vi "GFITS_CollectHeaders.vi"(2 "Database RefNum in":T1, 7 "Keywords":string[][](array[string]), 9 "extension":i16=-1, 11 "error in (no error)":errorcluster, 13 "nd queue":bool) -> (8 "headers":string[][](table), 15 "error out":errorcluster)   [LabVIEW 2016]
uses:
  GFITS_datatypesctl.ctl
  DBSHAND/private/vis/DatabaseHand_RefNum.ctl
panel:
  in  "Types":T2={"TBIT"=1, "TBYTE"=11, "TSTRING"=16, "TSHORT"=21, "TLONG"=41, "TFLOAT"=42, "TDOUBLE"=82, "TCOMPLEX"=83, "TDBLCOMPLEX"=163, "TUINT"=30, "TUSHORT"=20, "TULONG"=40, "TINT"=31, "TSBYTE"=12, "TLONGLONG"=81, "TLOGICAL"=14}
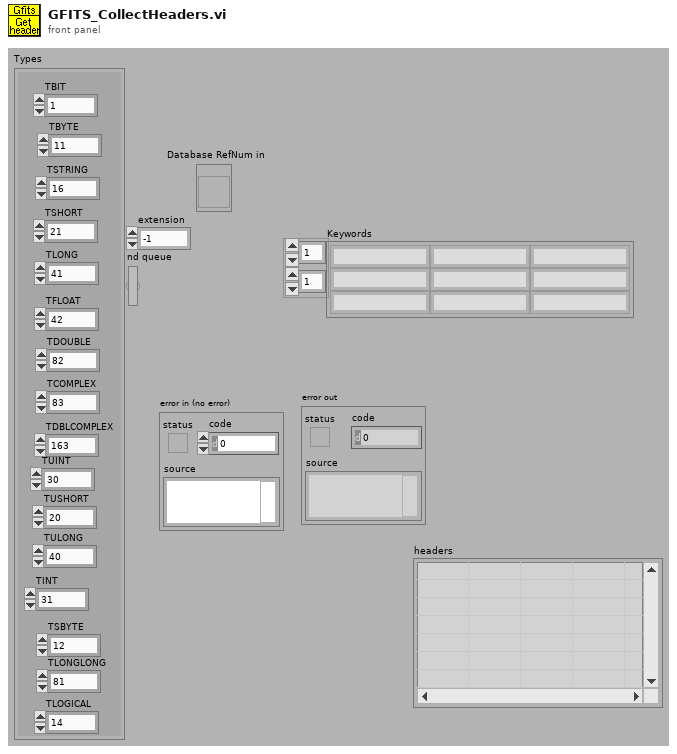
[diagram p1: front panel]
types:
  T1 = typedef "DatabaseHand_RefNum.ctl" = refnum<vi>
  T2 = typedef "GFITS_datatypesctl.ctl" = cluster{"TBIT":i32, "TBYTE":i32, "TSTRING":i32, "TSHORT":i32, "TLONG":i32, "TFLOAT":i32, "TDOUBLE":i32, "TCOMPLEX":i32, "TDBLCOMPLEX":i32, "TUINT":i32, "TUSHORT":i32, "TULONG":i32, "TINT":i32, "TSBYTE":i32, "TLONGLONG":i32, "TLOGICAL":i32}
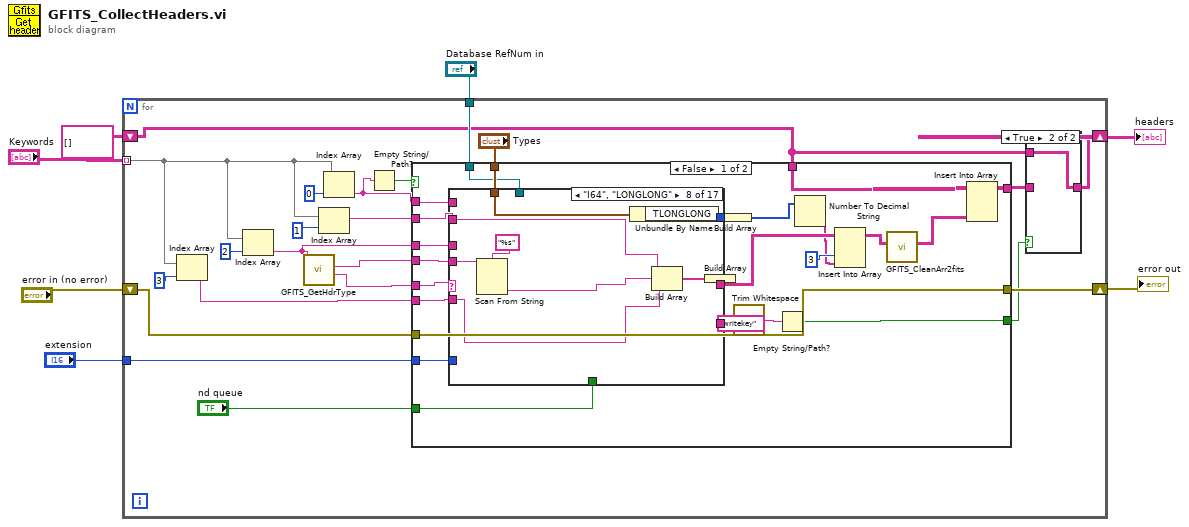
[diagram p0: block diagram]
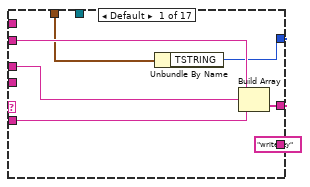
[diagram p3: hidden frame]
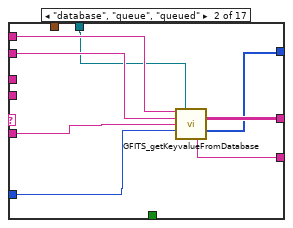
[diagram p4: hidden frame]
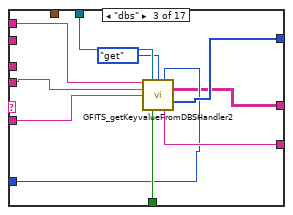
[diagram p5: hidden frame]
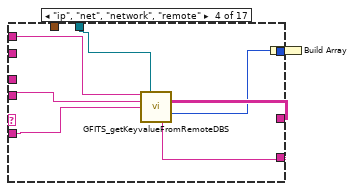
[diagram p6: hidden frame]
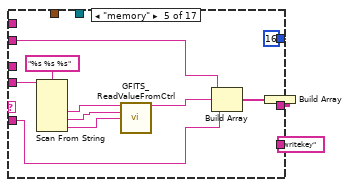
[diagram p7: hidden frame]
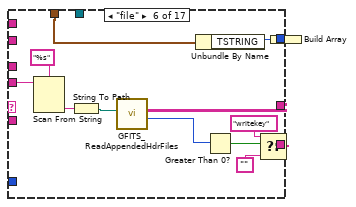
[diagram p8: hidden frame]
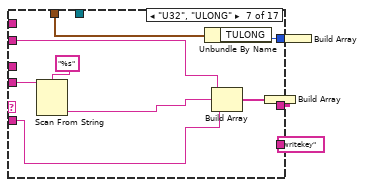
[diagram p9: hidden frame]
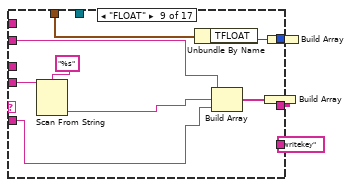
[diagram p10: hidden frame]
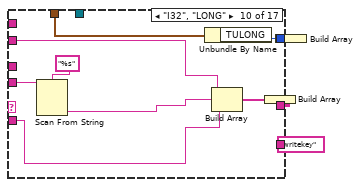
[diagram p11: hidden frame]
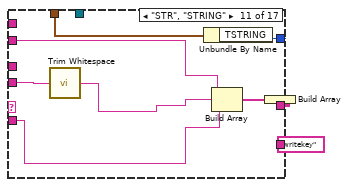
[diagram p12: hidden frame]
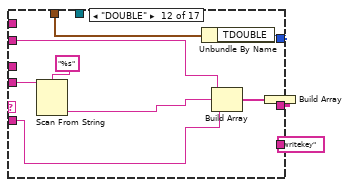
[diagram p13: hidden frame]
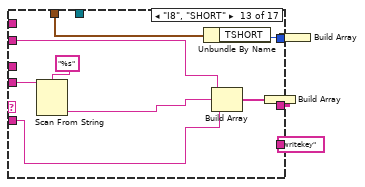
[diagram p14: hidden frame]
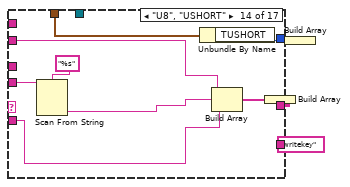
[diagram p15: hidden frame]
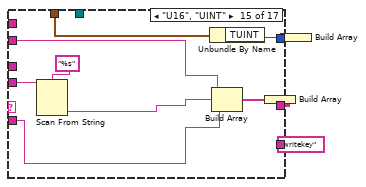
[diagram p16: hidden frame]
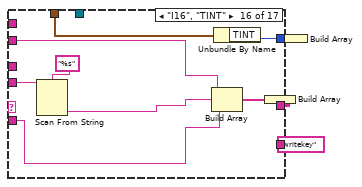
[diagram p17: hidden frame]
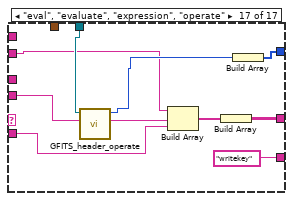
[diagram p18: hidden frame]
diagram:
  n1 = for {
    tunnel: "Keywords" -> [w24] mode=indexing
    shift-right: [w15] -> w6
    shift-left: "error in (no error)" -> [w19]
    tunnel: "Database RefNum in" -> [w18]
    shift-right: [w9] -> w2
    shift-left: string[][] [] -> [w8]
    tunnel: "extension" -> [w13]
    n2 = Index Array(array=w24, index=3 ("Array Index")) -> (element=w25:string)
    n3 = Index Array(array=w24, index=2 ("Array Index")) -> (element=w14:string)
    n4 = call "GFITS_GetHdrType.vi"("keyval"=w14) -> ("type"=w17:string, "keyval out"=w16:string)  [unwired: 9 out]
    n5 = Index Array(array=w24, index=1 ("Array Index")) -> (element=w26:string)
    n6 = Index Array(array=w24, index=0 ("Index")) -> (element=w22:string)
    n7 = Empty String/Path?(string/path=w22) -> (empty?=w21:bool)
    n8 = case shown="False" w21 {
      selector: w21 -> [_ w234]
      tunnel: w26 -> [w52 _]
      tunnel: w25 -> [w49 _]
      tunnel: w17 -> [w50 _]
      tunnel: w16 -> [w51 _]
      tunnel: w22 -> [w53 _]
      tunnel: "Types" -> [w48 _]
      tunnel: [w46 w236] -> w15
      tunnel: w19 -> [w46 w236]
      tunnel: w18 -> [w47 _]
      tunnel: [w45 w235] -> w10
      tunnel: w8 -> [w44 w235]
      tunnel: w14 -> [w43 _]
      tunnel: w13 -> [w38 _]
      tunnel: "nd queue" -> [w37 _]
      tunnel: [w34 w234] -> w11
      frame False {
        n9 = case shown="\"I64\", \"LONGLONG\"" w50 {
          tunnel: w49 -> [w60 w69 w77 w83 w93 _ w121 w132 w143 w154 w166 w175 w186 w197 w208 w219 w227]
          tunnel: ["writekey" w70 w76 w88 "writekey" ("function to use") w103 "writekey" ("function to use") "writekey" ("function to use") "writekey" ("function to use") "writekey" ("function to use") "writekey" ("function to use") "writekey" ("function to use") "writekey" ("function to use") "writekey" ("function to use") "writekey" ("function to use") "writekey" ("function to use") "writekey" ("function to use")] -> w36
          tunnel: [w57 w64 w74 w81 w89 w102 w115 w126 w137 w148 w159 w169 w180 w191 w202 w213 w225] -> w40
          tunnel: w52 -> [w61 w66 _ _ w94 _ w122 w133 w144 w155 w167 w176 w187 w198 w209 w220 w226]
          tunnel: w51 -> [_ _ w78 w84 w101 w112 w125 w136 w147 w158 w161 w179 w190 w201 w212 w223 w230]
          tunnel: [w58 w68 w71 w87 w90 w106 w119 w130 w141 w152 w164 w173 w184 w195 w206 w217 w228] -> w42
          tunnel: w53 -> [_ w67 w79 w85 _ _ _ _ _ _ _ _ _ _ _ _ _]
          tunnel: w48 -> [w56 _ _ _ _ w114 w117 w128 w139 w150 w163 w171 w182 w193 w204 w215 _]
          tunnel: w47 -> [_ w65 w80 w82 _ _ _ _ _ _ _ _ _ _ _ _ w229]
          tunnel: w43 -> [w54 _ _ _ _ _ _ _ _ _ _ _ _ _ _ _ _]
          tunnel: w38 -> [_ w63 w72 _ _ _ _ _ _ _ _ _ _ _ _ _ _]
          tunnel: w37 -> [_ _ w73 _ _ _ _ _ _ _ _ _ _ _ _ _ _]
          frame Default {
            n10 = Unbundle By Name(w56) -> ("TSTRING"=w55:i32)
            n11 = Build Array(w61, w54, w60) -> (w59:string[])
            n12 = Build Array(w55) -> (w57:i32[])
            n13 = Build Array(w59) -> (w58:string[][])
          }
          frame "database", "queue", "queued" {
            n14 = call "GFITS_getKeyvalueFromDatabase.vi"("key name in header"=w67, "Database RefNum in"=w65, "Keyname"=w66, "comment"=w69, "extension"=w63) -> ("table out"=w68:string[][], "datatype"=w64:u16[], "function to use"=w70:string)  [unwired: 1 in, 7 out]
          }
          frame "dbs" {
            n15 = call "GFITS_getKeyvalueFromDBSHandler2.vi"("key name in header"=w79, "Database RefNum in"=w80, "action"=enum16{"get", "clear"}."get", "extension"=w72, "varname"=w78, "comment"=w77, "nd queue"=w73) -> ("table out"=w71:string[][], "datatype"=w74:u16[], "function to use"=w76:string)  [unwired: 2 in, 4 out]
          }
          frame "ip", "net", "network", "remote" {
            n16 = call "GFITS_getKeyvalueFromRemoteDBS.vi"("key name in header"=w85, "Database RefNum in"=w82, "varname"=w84, "comment"=w83) -> ("table out"=w87:string[][], "datatype"=w86:u16, "function to use"=w88:string)  [unwired: 2 in, 7 out]
            n17 = Build Array(w86) -> (w81:u16[])
          }
          frame "memory" {
            n18 = Scan From String(format string="%s %s %s" ("Format String"), input string=w101) -> (output 1=w99:string, output 2=w98:string, output 3=w97:string)  [unwired: 2 in, 6 out]
            n19 = call "GFITS_ReadValueFromCtrl.vi"("Vi name"=w99, "Control Name"=w98, "Type"=w97) -> ("Value"=w92:string)  [unwired: 1 in, 11 out]
            n20 = Build Array(w94, w92, w93) -> (w91:string[])
            n21 = Build Array(w91) -> (w90:string[][])
            n22 = Build Array(16 ("datatype")) -> (w89:i32[])
          }
          frame "file" {
            n23 = Scan From String(format string="%s", input string=w112) -> (output 1=w110:string)  [unwired: 2 in, 4 out]
            n24 = String To Path(string=w110) -> (path=w109:path)
            n25 = call "GFITS_ReadAppendedHdrFiles.vi"("Path"=w109) -> ("keywords found"=w108:i32, "Array"=w106:string[][])  [unwired: 1 in, 8 out]
            n26 = Unbundle By Name(w114) -> ("TSTRING"=w113:i32)
            n27 = Greater Than 0?(x=w108) -> (x > 0?=w107:bool)
            n28 = Select(t="writekey" ("function to use"), s=w107, f="") -> (s? t:f=w103:string)
            n29 = Build Array(w113) -> (w102:i32[])
          }
          frame "U32", "ULONG" {
            n30 = Scan From String(format string="%s" ("Format String"), input string=w125) -> (output 1=w118:string)  [unwired: 2 in, 4 out]
            n31 = Unbundle By Name(w117) -> ("TULONG"=w116:i32)
            n32 = Build Array(w122, w118, w121) -> (w120:string[])
            n33 = Build Array(w120) -> (w119:string[][])
            n34 = Build Array(w116) -> (w115:i32[])
          }
          frame "I64", "LONGLONG" {
            n35 = Scan From String(format string="%s" ("Format String"), input string=w136) -> (output 1=w129:string)  [unwired: 2 in, 4 out]
            n36 = Unbundle By Name(w128) -> ("TLONGLONG"=w127:i32)
            n37 = Build Array(w133, w129, w132) -> (w131:string[])
            n38 = Build Array(w131) -> (w130:string[][])
            n39 = Build Array(w127) -> (w126:i32[])
          }
          frame "FLOAT" {
            n40 = Scan From String(format string="%s" ("Format String"), input string=w147) -> (output 1=w140:string)  [unwired: 2 in, 4 out]
            n41 = Unbundle By Name(w139) -> ("TFLOAT"=w138:i32)
            n42 = Build Array(w144, w140, w143) -> (w142:string[])
            n43 = Build Array(w142) -> (w141:string[][])
            n44 = Build Array(w138) -> (w137:i32[])
          }
          frame "I32", "LONG" {
            n45 = Scan From String(format string="%s" ("Format String"), input string=w158) -> (output 1=w151:string)  [unwired: 2 in, 4 out]
            n46 = Unbundle By Name(w150) -> ("TULONG"=w149:i32)
            n47 = Build Array(w155, w151, w154) -> (w153:string[])
            n48 = Build Array(w153) -> (w152:string[][])
            n49 = Build Array(w149) -> (w148:i32[])
          }
          frame "STR", "STRING" {
            n50 = call <vilib>:"Trim Whitespace.vi"("string"=w161) -> ("trimmed string"=w160:string)  [unwired: 1 in]
            n51 = Unbundle By Name(w163) -> ("TSTRING"=w162:i32)
            n52 = Build Array(w167, w160, w166) -> (w165:string[])
            n53 = Build Array(w165) -> (w164:string[][])
            n54 = Build Array(w162) -> (w159:i32[])
          }
          frame "DOUBLE" {
            n55 = Scan From String(format string="%s" ("Format String"), input string=w179) -> (output 1=w172:string)  [unwired: 2 in, 4 out]
            n56 = Unbundle By Name(w171) -> ("TDOUBLE"=w170:i32)
            n57 = Build Array(w176, w172, w175) -> (w174:string[])
            n58 = Build Array(w174) -> (w173:string[][])
            n59 = Build Array(w170) -> (w169:i32[])
          }
          frame "I8", "SHORT" {
            n60 = Scan From String(format string="%s" ("Format String"), input string=w190) -> (output 1=w183:string)  [unwired: 2 in, 4 out]
            n61 = Unbundle By Name(w182) -> ("TSHORT"=w181:i32)
            n62 = Build Array(w187, w183, w186) -> (w185:string[])
            n63 = Build Array(w185) -> (w184:string[][])
            n64 = Build Array(w181) -> (w180:i32[])
          }
          frame "U8", "USHORT" {
            n65 = Scan From String(format string="%s" ("Format String"), input string=w201) -> (output 1=w194:string)  [unwired: 2 in, 4 out]
            n66 = Unbundle By Name(w193) -> ("TUSHORT"=w192:i32)
            n67 = Build Array(w198, w194, w197) -> (w196:string[])
            n68 = Build Array(w196) -> (w195:string[][])
            n69 = Build Array(w192) -> (w191:i32[])
          }
          frame "U16", "UINT" {
            n70 = Scan From String(format string="%s" ("Format String"), input string=w212) -> (output 1=w205:string)  [unwired: 2 in, 4 out]
            n71 = Unbundle By Name(w204) -> ("TUINT"=w203:i32)
            n72 = Build Array(w209, w205, w208) -> (w207:string[])
            n73 = Build Array(w207) -> (w206:string[][])
            n74 = Build Array(w203) -> (w202:i32[])
          }
          frame "I16", "TINT" {
            n75 = Scan From String(format string="%s" ("Format String"), input string=w223) -> (output 1=w216:string)  [unwired: 2 in, 4 out]
            n76 = Build Array(w220, w216, w219) -> (w218:string[])
            n77 = Unbundle By Name(w215) -> ("TINT"=w214:i32)
            n78 = Build Array(w218) -> (w217:string[][])
            n79 = Build Array(w214) -> (w213:i32[])
          }
          frame "eval", "evaluate", "expression", "operate" {
            n80 = call "GFITS_header_operate.vi"("expression"=w230, "Database RefNum in"=w229) -> ("value"=w231:string, "numeric data type"=w232:i32)  [unwired: 8 out]
            n81 = Build Array(w226, w231, w227) -> (w233:string[])
            n82 = Build Array(w233) -> (w228:string[][])
            n83 = Build Array(w232) -> (w225:i32[])
          }
        }
        n84 = call <vilib>:"Trim Whitespace.vi"("string"=w36) -> ("trimmed string"=w35:string)  [unwired: 1 in]
        n85 = Empty String/Path?(string/path=w35) -> (empty?=w34:bool)
        n86 = Number To Decimal String(number=w40) -> (decimal integer string=w39:string[])  [unwired: 1 out]
        n87 = Insert Into Array(array=w42, index (col)=3 ("disabled index (col)"), new element=w39) -> (w33:string[][])  [unwired: 1 in]
        n88 = call "GFITS_CleanArr2fits.vi"("array"=w33) -> ("array out"=w32:string[][])  [unwired: 10 out]
        n89 = Insert Into Array(array=w44, new element=w32) -> (w45:string[][])  [unwired: 2 in]
      }
      frame True {
      }
    }
    n90 = case shown="True" w11 {
      tunnel: w10 -> [w30 _]
      tunnel: [w30 w31] -> w9
      tunnel: w8 -> [_ w31]
      frame False {
      }
      frame True {
      }
    }
  }
  "error out" <- w6
  "headers" <- w2
